vi "FGV_PSP - VRM Action Status.vi"(4 "error in":errorcluster, 6 "Function":enum16{"write", "read"}(ring), 7 "VRM Actions":T1) -> (0 "error out":errorcluster, 3 "VRM Actions":T1)   [LabVIEW 2016]
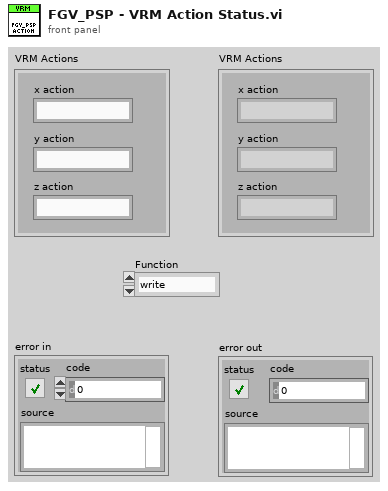
[diagram p1: front panel]
types:
  T1 = cluster{"x action":string, "y action":string, "z action":string}
  T2 = cluster{"[0]":string, "[1]":string, "[2]":string}
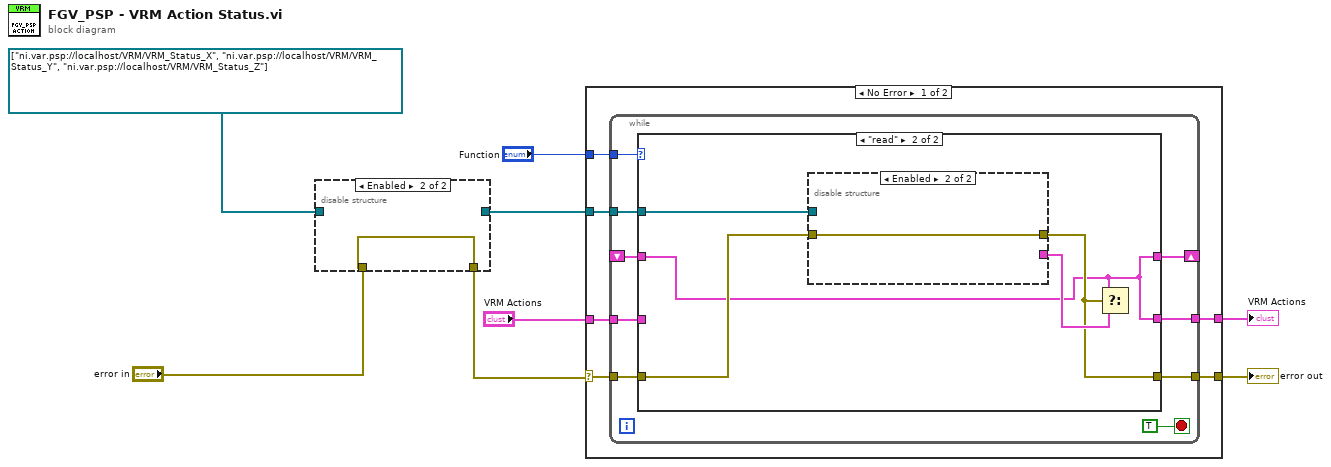
[diagram p0: block diagram]
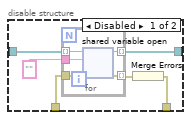
[diagram p2: hidden frame]
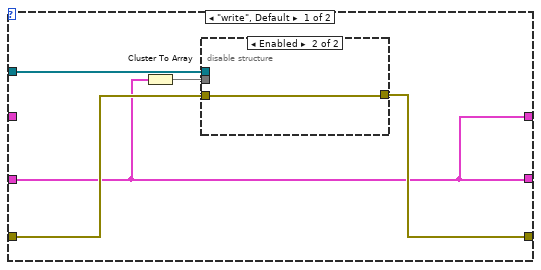
[diagram p3: hidden frame]
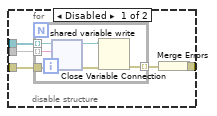
[diagram p4: hidden frame]
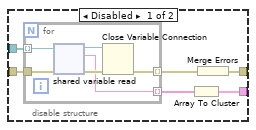
[diagram p5: hidden frame]
diagram:
  n1 = disable-structure shown="Enabled" {
    disable-tunnel: [w14 _] -> w6
    disable-tunnel: "error in" -> [w12 w20]
    disable-tunnel: refnum<k21>[] ["ni.var.psp://localhost/VRM/VRM_Status_X", "ni.var.psp://localhost/VRM/VRM_Status_Y", "ni.var.psp://localhost/VRM/VRM_Status_Z"] -> [w10 _]
    disable-tunnel: [w9 w20] -> w1
    frame Disabled {
      n2 = for {
        tunnel: [w19] -> w14 mode=indexing
        tunnel: w10 -> [w18] mode=indexing
        tunnel: [w17] -> w13 mode=indexing
        tunnel: w12 -> [w16]
        tunnel: "" -> [w15]
        n3 = shared-variable-open(w18, w16, w15) -> (w19:refnum<k21>, w17:errorcluster)  [unwired: 1 in]
      }
      n4 = Merge Errors(w13) -> (w9:errorcluster)
    }
    frame Enabled {
    }
  }
  n5 = case shown="No Error" w1 {
    selector: w1 -> [w26 w72]
    tunnel: [w25 w72] -> w8
    tunnel: [w24 w71] -> w4
    tunnel: "Function" -> [w23 _]
    tunnel: w6 -> [w22 _]
    tunnel: "VRM Actions" -> [w21 w71]
    frame No Error {
      n6 = while {
        shift-right: [w30] -> _
        shift-left: _ -> [w29]
        tunnel: w26 -> [w34]
        tunnel: [w33] -> w25
        tunnel: [w32] -> w24
        tunnel: w23 -> [w31]
        tunnel: w22 -> [w28]
        tunnel: w21 -> [w27]
        stop <- TRUE stop-if-true
        n7 = case shown="\"read\"" w31 {
          tunnel: w34 -> [w40 w56]
          tunnel: [w37 w54] -> w33
          tunnel: [w36 w53] -> w32
          tunnel: [w36 w53] -> w30
          tunnel: w29 -> [_ w53]
          tunnel: w28 -> [w39 w57]
          tunnel: w27 -> [w36 _]
          frame "write", Default {
            n8 = Cluster To Array(cluster=w36) -> (array=w38:string[])
            n9 = disable-structure shown="Enabled" {
              disable-tunnel: w40 -> [w44 w52]
              disable-tunnel: w39 -> [w43 _]
              disable-tunnel: w38 -> [w42 _]
              disable-tunnel: [w41 w52] -> w37
              frame Disabled {
                n10 = for {
                  tunnel: [w50] -> w45 mode=indexing
                  tunnel: w44 -> [w48]
                  tunnel: w43 -> [w47] mode=indexing
                  tunnel: w42 -> [w46] mode=indexing
                  n11 = shared-variable-write(w47, w48, w46) -> (w49:refnum<k21>, w51:errorcluster)
                  n12 = Close Variable Connection(8:w51, 11:w49) -> (0:w50:errorcluster)
                }
                n13 = Merge Errors(w45) -> (w41:errorcluster)
              }
              frame Enabled {
              }
            }
          }
          frame "read" {
            n14 = disable-structure shown="Enabled" {
              disable-tunnel: w57 -> [w62 _]
              disable-tunnel: w56 -> [w61 w70]
              disable-tunnel: [w59 _] -> w55
              disable-tunnel: [w58 w70] -> w54
              frame Disabled {
                n15 = for {
                  tunnel: [w67] -> w63 mode=indexing
                  tunnel: w62 -> [w66] mode=indexing
                  tunnel: w61 -> [w65]
                  tunnel: [w64] -> w60 mode=indexing
                  n16 = shared-variable-read(w66, w65) -> (w69:refnum<k21>, w68:errorcluster, w64:string)  [unwired: 1 out]
                  n17 = Close Variable Connection(8:w68, 11:w69) -> (0:w67:errorcluster)
                }
                n18 = Array To Cluster(array=w60) -> (cluster=w59:T2)
                n19 = Merge Errors(w63) -> (w58:errorcluster)
              }
              frame Enabled {
              }
            }
            n20 = Select(t=w53, s=w54, f=w55) -> ()  [unwired: 1 out]
          }
        }
      }
    }
    frame Error {
    }
  }
  "error out" <- w8
  "VRM Actions" <- w4
